vi "DriveExecute.vi"(8 "error in (no error)":errorcluster) -> (0 "error out":errorcluster)   [LabVIEW 2023]
doc: "Execute for Drie\n\nClosed control loop for drive\n\ninput: \n error in (cluster)\n\noutput:\n error out (cluster)"
uses:
  <vilib>/Rock Robotics/WPI/ThirdParty/JAS_Junk/TrajLib/Rotation2d_CreateAngleDegrees.vi
  <vilib>/Rock Robotics/WPI/ThirdParty/JAS_Junk/TrajLib/SwerveModuleState_New.vi
  <vilib>/Rock Robotics/WPI/ThirdParty/JAS_Junk/TrajLib/VI/SwerveModulePosition_New.vi
  <vilib>/Rock Robotics/WPI/ThirdParty/JAS_Junk/TrajLib/MathUtil_InputModulus.vi
  <vilib>/Rock Robotics/WPI/ThirdParty/JAS_Junk/TrajLib/Conv_Feet_Meters.vi
  DriveGetModuleRef.vi
  <vilib>/Rock Robotics/WPI/ThirdParty/JAS_Junk/TrajLib/LinearFilter_ResetToValue.vi
  <vilib>/Rock Robotics/WPI/ThirdParty/JAS_Junk/TrajLib/LinearFilter_Calculate.vi
  <vilib>/Rock Robotics/WPI/ThirdParty/JAS_Junk/TrajLib/Conv_Deg_Radians.vi
  <vilib>/Rock Robotics/WPI/ThirdParty/JAS_Junk/TrajLib/Rotation2d_CreateAngle.vi
  DriveGlobal.vi
  <vilib>/Rock Robotics/WPI/ThirdParty/JAS_Junk/TrajLib/LinearFilter_MovingAverage.vi
  <vilib>/Rock Robotics/WPI/ThirdParty/JAS_Junk/TrajLib/LinearFilter_LowPassBW1.vi
  <vilib>/Rock Robotics/WPI/ThirdParty/JAS_Junk/TrajLib/LinearFilter_LowPassBW2.vi
  <vilib>/Rock Robotics/WPI/ThirdParty/JAS_Junk/TrajLib/LinearFilter_HighPassBW1.vi
  <vilib>/Rock Robotics/WPI/ThirdParty/JAS_Junk/TrajLib/LinearFilter_HighPassBW2.vi
  <vilib>/Rock Robotics/WPI/ThirdParty/Phoenix-LabVIEW/CANCoder/CTRE_Phoenix_CANcoder_RefNumRegistryGet.vi
  <vilib>/Rock Robotics/WPI/MotorControl/WPI_MotorControlRefNum Registry Get.vi
  <vilib>/Rock Robotics/WPI/ThirdParty/REV Robotics/REVLib/SubVI/Deprecated/Spark MAX Get Sensor Position.vi
  <vilib>/Rock Robotics/WPI/ThirdParty/REV Robotics/REVLib/SubVI/Deprecated/Spark MAX Get Sensor Velocity.vi
  <vilib>/Rock Robotics/WPI/ThirdParty/Phoenix-LabVIEW/CANCoder/CTRE_Phoenix_CANcoder_GetPolymorphic.vi
  <vilib>/Rock Robotics/WPI/ThirdParty/Phoenix-LabVIEW/CANCoder/Get/CTRE_Phoenix_CANcoder_GetSensorData.vi
  <vilib>/Rock Robotics/Network Tables/NT Write Value.vi
  <vilib>/Rock Robotics/Network Tables/NT Write Number.vi
  <vilib>/Rock Robotics/WPI/ThirdParty/JAS_Junk/TrajLib/Trajectory_Library.lvlib
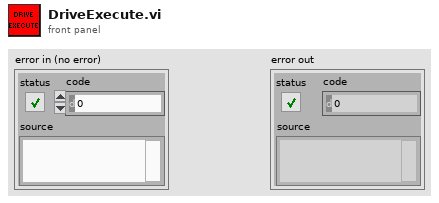
[diagram p1: front panel]
types:
  T1 = enum16{"Moving Average", "Low Pass 1st Order Butterworth", "Low Pass 2nd Order Butterworth", "High Pass 1st Order Butterworth", "High Pass 2nd Order Butterworth"}
  T2 = typedef "Trajectory_Library.lvlib/CHASSIS_SPEEDS.ctl" = cluster{"vX":dbl, "vY":dbl, "vOmega":dbl}
  T3 = typedef "ADIS16470 Device Reference.ctl" = cluster{"DevStatus":errorcluster, "Hardware Config":T4, "Calibration Complete":refnum<notifier>, "Status Reference":refnum<data-value>, "Data Reference":refnum<data-value>, "Sychronous Process VI":T8, "Cmd FIFO":refnum<k33>, "Source":T9, "Data FIFO":refnum<k33>, "Calibration Time (ms)":u32, "Data Reference":refnum<data-value>}
  T4 = typedef "ADIS16470 Hardware Configuration.ctl" = cluster{"SPI Clock Rate (Hz)":dbl, "IMU SPI Mode (3)":T5, "IMU Reset Pin":T6, "IMU SPI Bus":T7, "IMU Data Ready Pin":T6, "Stall Config":cluster{"Pow2BytesPerRead":u8, "StallTicks":u16, "CsToSclkTicks":u8}}
  T5 = typedef "WPI_SPIMode.ctl" = enum16{"Mode 0 (Clk Idle Low,Sample on Leading)", "Mode 1 (Clk Idle Low,Sample on Trailing)", "Mode 2 (Clk Idle High,Sample on Leading)", "Mode 3 (Clk Idle High,Sample on Trailing)"}
  T6 = typedef "FPGA_DIOChannel.ctl" = enum8{"DIO 0", "DIO 1", "DIO 2", "DIO 3", "DIO 4", "DIO 5", "DIO 6", "DIO 7", "DIO 8", "DIO 9", "DIO MXP 0", "DIO MXP 1", "DIO MXP 2", "DIO MXP 3", "DIO MXP 4", "DIO MXP 5", "DIO MXP 6", "DIO MXP 7", "DIO MXP 8", "DIO MXP 9", "DIO MXP 10", "DIO MXP 11", "DIO MXP 12", "DIO MXP 13", "DIO MXP 14", "DIO MXP 15", "SPI Port CS1", "SPI Port CS2", "SPI Port CS3", "SPI Port MISO", "SPI Port MOSI", "Invalid"}
  T7 = typedef "spi_bus.ctl" = enum16{"SPI On-Board, CS0", "SPI On-Board, CS1", "SPI On-Board, CS2", "SPI On-Board, CS3", "SPI MXP", "Invalid"}
  T8 = typedef "ADIS16470 Process.ctl" = refnum<vi>
  T9 = typedef "FPGA_CounterEncoderSourceConvertionLVSourceType.ctl" = cluster{"DevStatus":errorcluster, "AnalogTriggerMode?":bool, "DigitalMode":cluster{"DIO Channel":T10}, "AnalogTriggerMode":cluster{"AnalogTriggerIndex":T11, "OutputType":T12}}
  T10 = typedef "FPGA_DIODigitalSourceChannel.ctl" = enum8{"DIO 0", "DIO 1", "DIO 2", "DIO 3", "DIO 4", "DIO 5", "DIO 6", "DIO 7", "DIO 8", "DIO 9", "DIO MXP 0", "DIO MXP 1", "DIO MXP 2", "DIO MXP 3", "DIO MXP 4", "DIO MXP 5", "DIO MXP 6", "DIO MXP 7", "DIO MXP 8", "DIO MXP 9", "DIO MXP 10", "DIO MXP 11", "DIO MXP 12", "DIO MXP 13", "DIO MXP 14", "DIO MXP 15", "SPI Port CS1", "SPI Port CS2", "SPI Port CS3", "SPI Port MISO", "SPI Port MOSI", "Disabled"}
  T11 = typedef "FPGA_AnalogTriggerIndex.ctl" = enum8{"Trig 0", "Trig 1", "Trig 2", "Trig 3", "Trig 4", "Trig 5", "Trig 6", "Trig 7", "Invalid"}
  T12 = typedef "FPGA_AnalogTriggerOutType.ctl" = enum16{"InWindow", "TriggerState", "Rising", "Falling"}
  T13 = typedef "Trajectory_Library.lvlib/SWERVE_DRIVE_KINEMATICS.ctl" = cluster{"NumModules":i32, "InverseKinematics":T14, "ForwardKinematics":T14, "Modules":T15[], "PrevCoR":T15, "SavedModuleStates":T16[]}
  T14 = typedef "NI_Matrix.lvlib/RealMatrix.ctl" = dbl[][]
  T15 = typedef "Trajectory_Library.lvlib/TRANSLATION2D.ctl" = cluster{"X":dbl, "Y":dbl}
  T16 = typedef "Trajectory_Library.lvlib/SWERVE_DRIVE_MODULE_STATE.ctl" = cluster{"Speed":dbl, "Angle":T17}
  T17 = typedef "Trajectory_Library.lvlib/ROTATION2D.ctl" = cluster{"VALUE":dbl, "COS":dbl, "SIN":dbl}
  T18 = typedef "Trajectory_Library.lvlib/SWERVE_DRIVE_MODULE_POSITION.ctl" = cluster{"Distance":dbl, "Angle":T17, "P":bool}
  T19 = typedef "ADIS16470 Data.ctl" = cluster{"XAngle":dbl, "YAngle":dbl, "ZAngle":dbl}
  T20 = typedef "ADIS16470 Status.ctl" = cluster{"Calibrated?":bool, "IMU Detected?":bool}
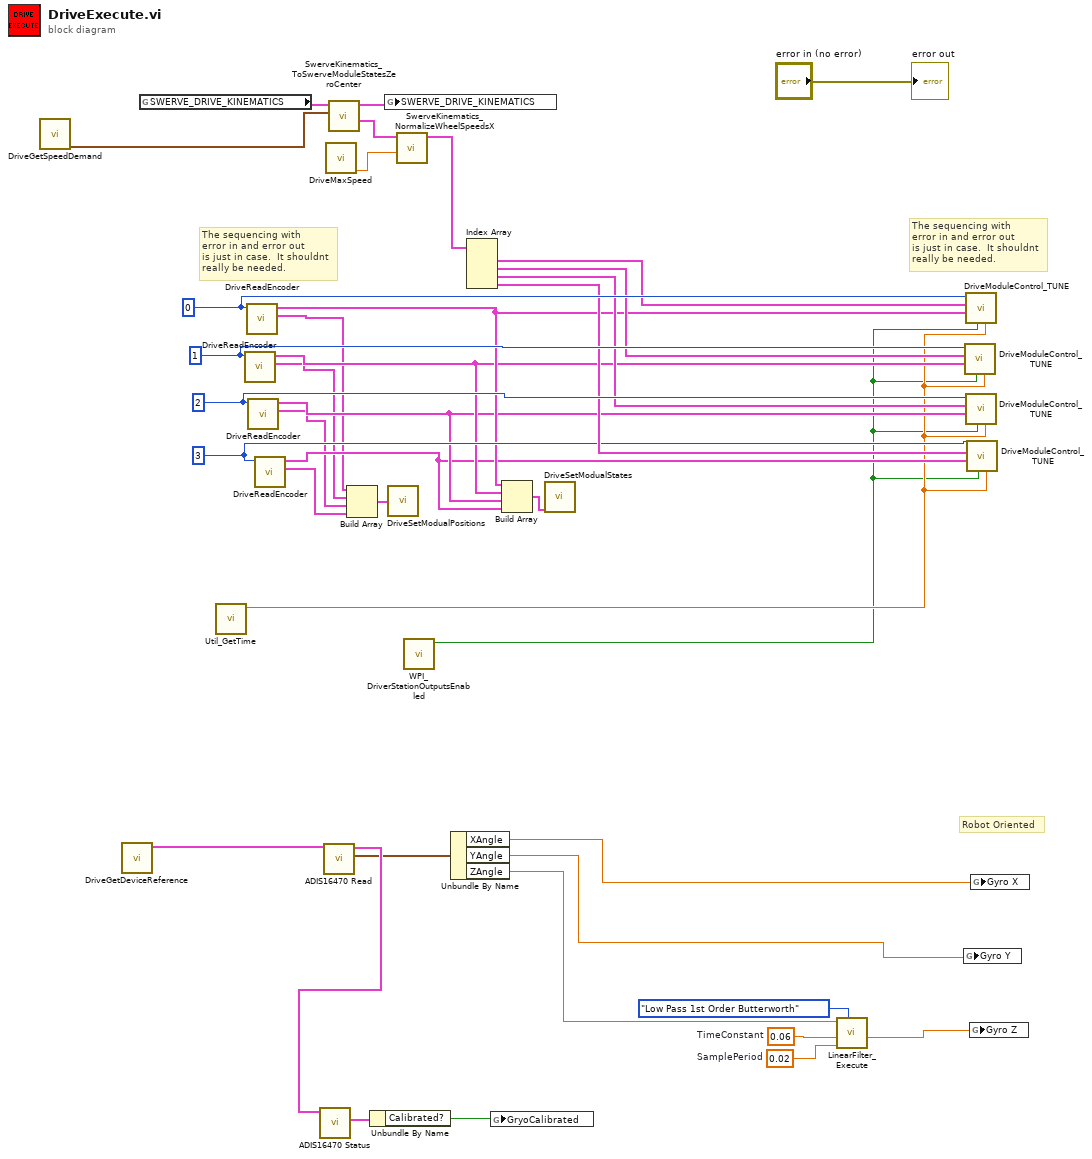
[diagram p0: block diagram]
diagram:
  w17 = 0.02  # SamplePeriod
  w16 = 0.06  # TimeConstant
  w35 = 0 ("ModualNamePrefix")
  w34 = 1 ("ModualNamePrefix")
  w33 = 2 ("ModualNamePrefix")
  w28 = 3 ("ModualNamePrefix")
  # "Robot Oriented"
  # "The sequencing with\nerror in and error out\nis just in case.  It shouldnt\nreally be needed."
  # "The sequencing with\nerror in and error out\nis just in case.  It shouldnt\nreally be needed."
  n1 = call "DriveGetSpeedDemand.vi"() -> ("ChassisSpeedDemand"=w37:T2)  [unwired: 8 in, 3 out]
  n2 = call "DriveGetDeviceReference.vi"() -> ("ADIS16470DevRef out"=w14:T3)  [unwired: 11 in]
  n3 = global read "DriveGlobal.vi" "SWERVE_DRIVE_KINEMATICS"() -> (w38:T13)
  n4 = call <vilib>:"Util_GetTime.vi"() -> ("FPGA_Time_Seconds"=w2:dbl)  [unwired: 9 in, 2 out]
  n5 = call "DriveReadEncoder.vi"("ModualNamePrefix"=w34) -> ("SWERVE_DRIVE_MODULE_POSITION"=w22:T18, "SWERVE_DRIVE_MODULE_STATE"=w26:T16)  [unwired: 8 in, 1 out]
  n6 = call "DriveReadEncoder.vi"("ModualNamePrefix"=w35) -> ("SWERVE_DRIVE_MODULE_POSITION"=w23:T18, "SWERVE_DRIVE_MODULE_STATE"=w27:T16)  [unwired: 8 in, 1 out]
  n7 = call "DriveReadEncoder.vi"("ModualNamePrefix"=w33) -> ("SWERVE_DRIVE_MODULE_POSITION"=w21:T18, "SWERVE_DRIVE_MODULE_STATE"=w25:T16)  [unwired: 8 in, 1 out]
  n8 = call "DriveReadEncoder.vi"("ModualNamePrefix"=w28) -> ("SWERVE_DRIVE_MODULE_POSITION"=w20:T18, "SWERVE_DRIVE_MODULE_STATE"=w24:T16)  [unwired: 8 in, 1 out]
  n9 = call <vilib>:"ADIS16470 Read.vi"("ADIS16470DevRef"=w14) -> ("ADIS16470 Value"=w10:T19, "ADIS16470DevRef"=w11:T3)  [unwired: 7 in, 2 out]
  n10 = call <vilib>:"ADIS16470 Status.vi"("ADIS16470DevRef"=w11) -> ("ADIS16470 Status"=w13:T20)  [unwired: 8 in, 2 out]
  n11 = call "DriveMaxSpeed.vi"() -> ("Max Speed (m/sec)"=w4:dbl)  [unwired: 10 in, 1 out]
  n12 = call <vilib>:"SwerveKinematics_ToSwerveModuleStatesZeroCenter.vi"("ChassisSpeeds"=w37, "in SWERVE_DRIVE_KINEMATICS"=w38) -> ("ModuleStates"=w5:T16[], "out SWERVE_DRIVE_KINEMATICS"=w36:T13)  [unwired: 8 in]
  n13 = Build Array(w23, w22, w21, w20) -> (w18:T18[])
  n14 = Unbundle By Name(w13) -> ("Calibrated?"=w12:bool)
  n15 = global write "DriveGlobal.vi" "SWERVE_DRIVE_KINEMATICS"(w36) -> ()
  n16 = call "DriveSetModualPositions.vi"("Swerve_Drive_Modual_Position"=w18) -> ()  [unwired: 11 in]
  n17 = call <vilib>:"SwerveKinematics_NormalizeWheelSpeedsX.vi"("AttainableMaxSpeed"=w4, "in WheelStates"=w5) -> ("out WheelStates"=w3:T16[])  [unwired: 9 in]
  n18 = call <vilib>:"WPI_DriverStationOutputsEnabled.vi"() -> ("OutputsEnabled?"=w1:bool)  [unwired: 10 in, 1 out]
  n19 = Unbundle By Name(w10) -> ("XAngle"=w8:dbl, "YAngle"=w7:dbl, "ZAngle"=w9:dbl)
  n20 = Index Array(array=w3) -> (element #1=w29:T16, element #2=w32:T16, element #3=w31:T16, element #4=w30:T16)  [unwired: 4 in]
  n21 = global write "DriveGlobal.vi" "GryoCalibrated"(w12) -> ()
  n22 = Build Array(w27, w26, w25, w24) -> (w19:T16[])
  n23 = call "DriveSetModualStates.vi"("Swerve__Drive_Modual_States"=w19) -> ()  [unwired: 11 in]
  n24 = call <vilib>:"LinearFilter_Execute.vi"("Filter Type"=T1."Low Pass 1st Order Butterworth", "SamplePeriod"=w17, "TimeConstant"=w16, "Input"=w9) -> ("Output"=w6:dbl)  [unwired: 6 in, 1 out]
  n25 = global write "DriveGlobal.vi" "Gyro Y"(w7) -> ()
  n26 = call "DriveModuleControl_TUNE.vi"("Time"=w2, "OutputsEnabled"=w1, "Actual State"=w26, "Desired State"=w32, "ModualNamePrefix"=w34) -> ()  [unwired: 6 in, 1 out]
  n27 = call "DriveModuleControl_TUNE.vi"("Time"=w2, "OutputsEnabled"=w1, "Actual State"=w27, "Desired State"=w29, "ModualNamePrefix"=w35) -> ()  [unwired: 6 in, 1 out]
  n28 = call "DriveModuleControl_TUNE.vi"("Time"=w2, "OutputsEnabled"=w1, "Actual State"=w25, "Desired State"=w31, "ModualNamePrefix"=w33) -> ()  [unwired: 6 in, 1 out]
  n29 = call "DriveModuleControl_TUNE.vi"("Time"=w2, "OutputsEnabled"=w1, "Actual State"=w24, "Desired State"=w30, "ModualNamePrefix"=w28) -> ()  [unwired: 6 in, 1 out]
  n30 = global write "DriveGlobal.vi" "Gyro Z"(w6) -> ()
  n31 = global write "DriveGlobal.vi" "Gyro X"(w8) -> ()
  "error out" <- "error in (no error)"
